vi "Write Command.vi"(6 "wait for reply (T)":bool=TRUE, 8 "error in (no error)":errorcluster, 10 "Command":string, 11 "Module ID":i32=-1) -> (0 "error out":errorcluster, 1 "timed out?":bool, 2 "Reply Payload":T1)   [LabVIEW 2017, in "SSH.lvlib"]
doc: "Writes out a command to the SSH client\n_____\nCreated using Delacor QMH Event Scripter 4.2.1.88."
uses:
  SSH.lvlib
  Write Command (Reply Payload)--cluster.ctl
  Write Command Argument--cluster.ctl
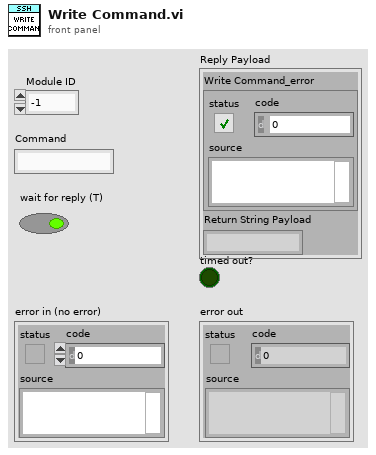
[diagram p1: front panel]
types:
  T1 = typedef "SSH.lvlib/Write Command (Reply Payload)--cluster.ctl" = cluster{"Write Command_error":errorcluster, "Return String Payload":string}
  T2 = typedef "SSH.lvlib/Write Command Argument--cluster.ctl" = cluster{"Module ID":i32, "Command":string, "Wait Notifier":refnum<notifier>, "wait for reply":bool}
  T3 = typedef "SSH.lvlib/Request Events--cluster.ctl" = cluster{"Stop Module":refnum<user-event>, "Show Panel":refnum<user-event>, "Hide Panel":refnum<user-event>, "Show Diagram":refnum<user-event>, "Get Module Execution Status":refnum<user-event>, "Write Command":refnum<user-event>, "Set Response Configuration":refnum<user-event>}
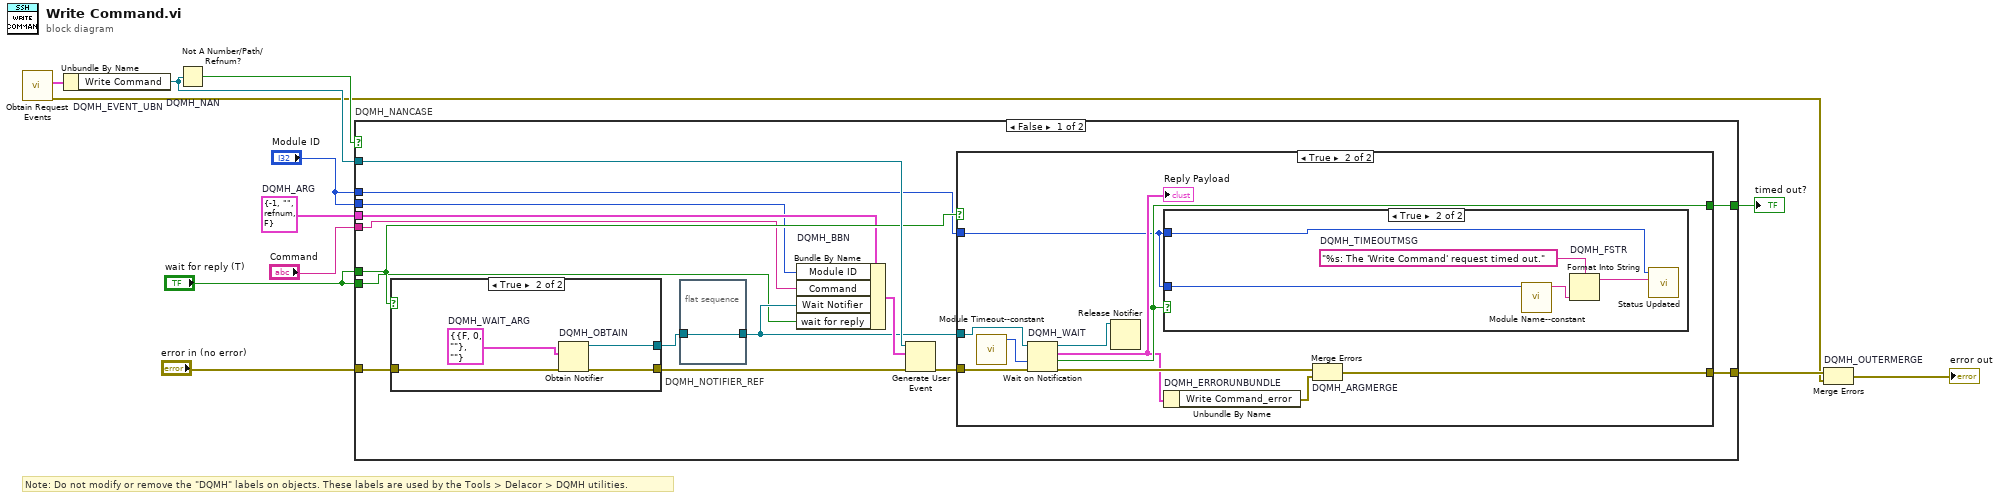
[diagram p0: block diagram]
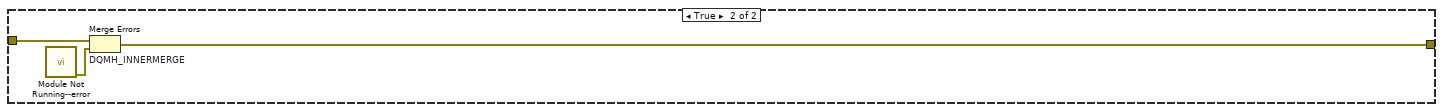
[diagram p5: hidden frame]
diagram:
  w6 = T2 {"Module ID"=-1, "Command"="", "Wait Notifier"=refnum, "wait for reply"=FALSE}  # DQMH_ARG
  # "Note: Do not modify or remove the \"DQMH\" labels on objects. These labels are used by the Tools > Delacor > DQMH utilities."
  n1 = call "Obtain Request Events.vi"() -> ("error out"=w2:errorcluster, "SSH Request Events"=w1:T3)  [unwired: 10 in]
  n2 = Unbundle By Name "DQMH_EVENT_UBN"(w1) -> ("Write Command"=w7:refnum<user-event>)
  n3 = Not A Number/Path/Refnum? "DQMH_NAN"(number/path/refnum=w7) -> (NaN/Path/Refnum?=w8:bool)
  n4 = case "DQMH_NANCASE" shown="False" w8 {
    tunnel: "error in (no error)" -> [w27 w52]
    tunnel: w7 -> [w25 _]
    tunnel: [w22 w51] -> w9
    tunnel: [w23 _] -> w11
    tunnel: "wait for reply (T)" -> [w20 _]
    tunnel: w6 -> [w17 _]
    tunnel: "Module ID" -> [w16 _]
    tunnel: "Command" -> [w15 _]
    tunnel: "Module ID" -> [w14 _]
    tunnel: "wait for reply (T)" -> [w13 _]
    frame False {
      n5 = case shown="True" w20 {
        tunnel: w27 -> [w45 w49]
        tunnel: [w45 w48] -> w24
        tunnel: [_ w46] -> w19
        frame False {
        }
        frame True {
          w47 = T1 {"Write Command_error"={"status"=FALSE, "code"=0, "source"=""}, "Return String Payload"=""}  # DQMH_WAIT_ARG
          n6 = Obtain Notifier "DQMH_OBTAIN"(notification data type=w47, error in (no error)=w49) -> (notifier out=w46:refnum<notifier>, error out=w48:errorcluster)  [unwired: 2 in, 1 out]
        }
      }
      n7 = flat-sequence "DQMH_NOTIFIER_REF" {
        tunnel: w19 -> [w28]
        tunnel: [w28] -> w18
        frame #0 {
        }
      }
      n8 = Bundle By Name "DQMH_BBN"(cluster=w17, "Module ID"=w16, "Command"=w15, "Wait Notifier"=w18, "wait for reply"=w13) -> (w21:T2)
      n9 = Generate User Event(user event=w25, event data cluster=w21, error in=w24) -> (error out=w26:errorcluster)  [unwired: 1 in, 1 out]
      n10 = case shown="True" w20 {
        tunnel: w26 -> [w29 w39]
        tunnel: w18 -> [_ w37]
        tunnel: [_ w35] -> w23
        tunnel: [w29 w34] -> w22
        tunnel: w14 -> [_ w30]
        frame False {
        }
        frame True {
          n11 = call "Module Timeout--constant.vi"() -> ("Module Timeout"=w31:i32)  [unwired: 11 in]
          n12 = Wait on Notification "DQMH_WAIT"(notifier=w37, timeout in ms (-1)=w31, error in (no error)=w39) -> (notifier out=w36:refnum<notifier>, notification=w32:T1, timed out?=w35:bool, error out=w38:errorcluster)  [unwired: 1 in]
          "Reply Payload" <- w32
          n13 = Release Notifier(notifier=w36) -> ()  [unwired: 2 in, 3 out]
          n14 = case shown="True" w35 {
            tunnel: w30 -> [_ w41]
            tunnel: w30 -> [_ w40]
            frame False {
            }
            frame True {
              w44 = "%s: The 'Write Command' request timed out."  # DQMH_TIMEOUTMSG
              n15 = call "Module Name--constant.vi"("Module ID"=w40) -> ("Module Name"=w43:string)  [unwired: 10 in]
              n16 = Format Into String "DQMH_FSTR"(format string=w44, w43) -> (resulting string=w42:string)  [unwired: 2 in, 1 out]
              n17 = call "Status Updated.vi"("Status"=w42, "Module ID"=w41) -> ()  [unwired: 9 in, 1 out]
            }
          }
          n18 = Unbundle By Name "DQMH_ERRORUNBUNDLE"(w32) -> ("Write Command_error"=w33:errorcluster)
          n19 = Merge Errors "DQMH_ARGMERGE"(w38, w33) -> (w34:errorcluster)
        }
      }
    }
    frame True {
      n20 = call "Module Not Running--error.vi"() -> ("error out"=w50:errorcluster)  [unwired: 11 in]
      n21 = Merge Errors "DQMH_INNERMERGE"(w52, w50) -> (w51:errorcluster)
    }
  }
  "timed out?" <- w11
  n22 = Merge Errors "DQMH_OUTERMERGE"(w9, w2) -> (→"error out":errorcluster)
